vi "FindThetas.vi"(0 "strip":T3 {"a (cm)" format="%.2f"; "h (cm)" format="%.2f"; "radius (cm)" format="%.2f"}, 1 "r values (cm)":T5 {"r5" format="%.2f"; "r4" format="%.2f"; "r3" format="%.2f"; "r2" format="%.2f"; "r1" format="%.2f"; "r0" format="%.2f"}, 3 "Case Number":i32, 4 "Location Tests":T1, 5 "P constants":T4 {"Dtemp" format="%.2f"; "B" format="%.2f"; "A" format="%.2f"; "thetaw" format="%.2f"; "phih" format="%.2f"; "r (cm)" format="%.2f"}, 6 "Variables":T2={"sound spd (cm/s)"=150000, "time step (s)"=1e-09} {"time step (s)" format="%.2e"}, 7 "P (cm)":cluster{"x":dbl, "y":dbl, "z":dbl}={"x"=1.0, "y"=-5.0, "z"=2.0} {"x" format="%.2f"; "z" format="%.2f"; "y" format="%.2f"}) -> (8 "d":dbl[](array[numeric]) format="%.2f", 9 "min/max r":cluster{"max":dbl, "min":dbl} {"min" format="%.2f"; "max" format="%.2f"}, 10 "h(r,t) offset":dbl[](graph), 11 "cap to wedge offset":i32, 12 "h(r,t)":dbl[](graph), 13 "wedge delay pts":i32, 14 "beta(t)/2":dbl[](array[numeric]) format="%.2f", 15 "cap delay pts":i32, 17 "rmin out":dbl format="%.2f", 18 "sigma":dbl[](array[numeric]) format="%.2f", 19 "slice coords":dbl[][](array[numeric]) format="%.4f")   [LabVIEW 2022 SP3]
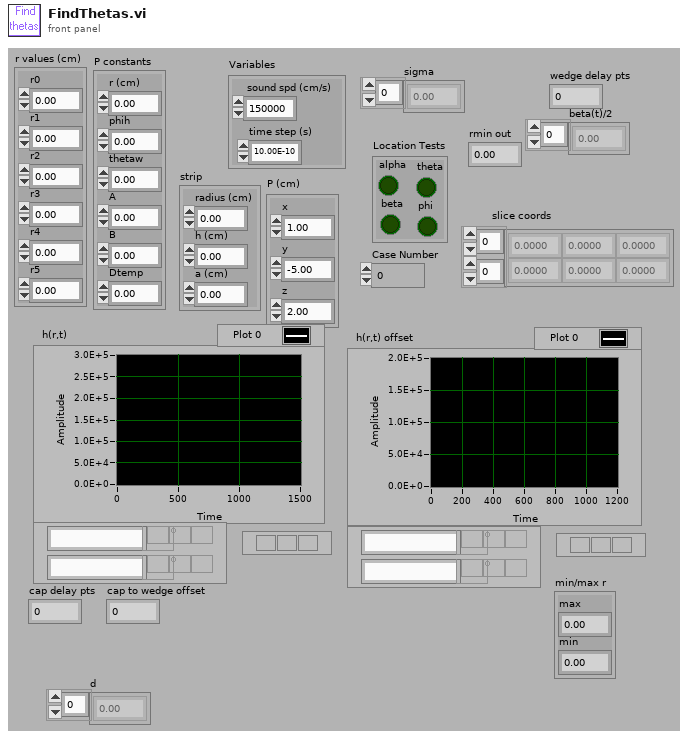
[diagram p1: front panel]
types:
  T1 = cluster{"alpha":bool, "beta":bool, "theta":bool, "phi":bool}
  T2 = cluster{"sound spd (cm/s)":i32, "time step (s)":sgl}
  T3 = cluster{"radius (cm)":dbl, "h (cm)":dbl, "a (cm)":dbl}
  T4 = cluster{"r (cm)":dbl, "phih":dbl, "thetaw":dbl, "A":dbl, "B":dbl, "Dtemp":dbl}
  T5 = cluster{"r0":dbl, "r1":dbl, "r2":dbl, "r3":dbl, "r4":dbl, "r5":dbl}
  T6 = cluster{"Number of rings":i32, "sound spd (cm/s)":i32, "z span (cm)":dbl, "z steps":i32, "y span (cm)":dbl, "y steps":i32, "time step (s)":sgl, "z":dbl, "y":dbl, "ref delay":dbl, "freq (MHz)":dbl, "cycles":i32}
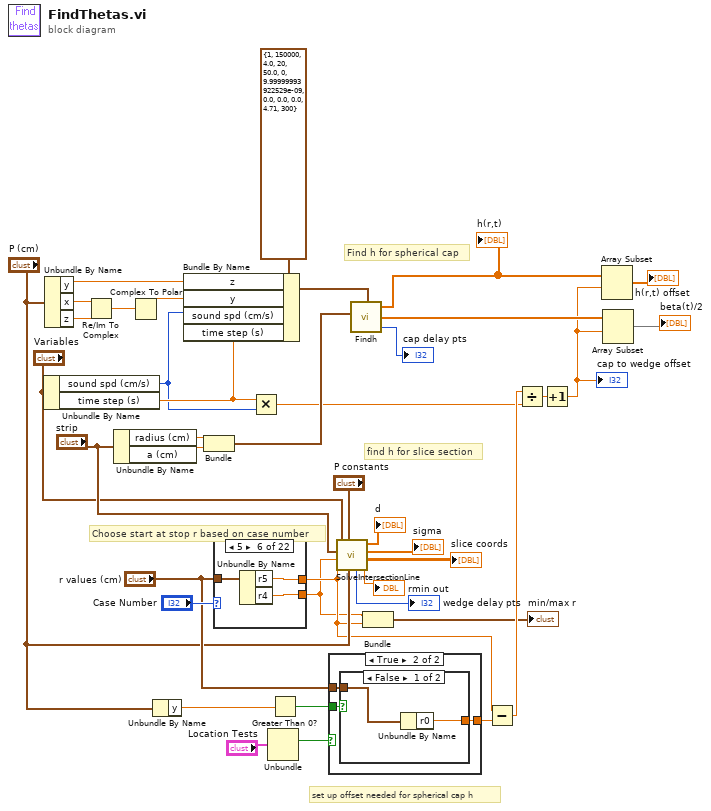
[diagram p0: block diagram]
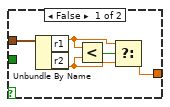
[diagram p2: hidden frame]
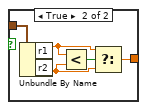
[diagram p3: hidden frame]
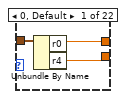
[diagram p4: hidden frame]
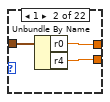
[diagram p5: hidden frame]
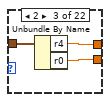
[diagram p6: hidden frame]
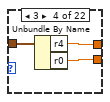
[diagram p7: hidden frame]
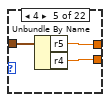
[diagram p8: hidden frame]
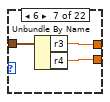
[diagram p9: hidden frame]
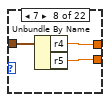
[diagram p10: hidden frame]
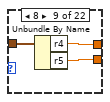
[diagram p11: hidden frame]
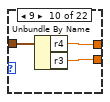
[diagram p12: hidden frame]
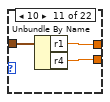
[diagram p13: hidden frame]
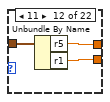
[diagram p14: hidden frame]
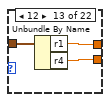
[diagram p15: hidden frame]
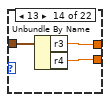
[diagram p16: hidden frame]
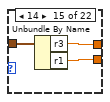
[diagram p17: hidden frame]
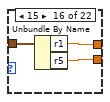
[diagram p18: hidden frame]
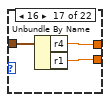
[diagram p19: hidden frame]
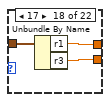
[diagram p20: hidden frame]
diagram:
  # "Find h for spherical cap"
  # "find h for slice section"
  # "set up offset needed for spherical cap h"
  # "Choose start at stop r based on case number"
  n1 = Unbundle By Name("Variables") -> ("sound spd (cm/s)"=w6:i32, "time step (s)"=w20:sgl)
  n2 = Unbundle By Name("P (cm)") -> ("y"=w17:dbl, "x"=w33:dbl, "z"=w32:dbl)
  n3 = Re/Im To Complex(1:w32, 2:w33) -> (0:w31:cdb)
  n4 = Unbundle By Name("strip") -> ("radius (cm)"=w36:dbl, "a (cm)"=w35:dbl)
  n5 = Complex To Polar(r * e^(i*theta)=w31) -> (r=w18:dbl)  [unwired: 1 out]
  n6 = Unbundle By Name("P (cm)") -> ("y"=w19:dbl)
  n7 = Bundle By Name(cluster=T6 {"Number of rings"=1, "sound spd (cm/s)"=150000, "z span (cm)"=4.0, "z steps"=20, "y span (cm)"=50.0, "y steps"=0, "time step (s)"=1e-08, "z"=0.0, "y"=0.0, "ref delay"=0.0, "freq (MHz)"=4.71, "cycles"=300} ("Variables in"), "z"=w17, "y"=w18, "sound spd (cm/s)"=w6, "time step (s)"=w20) -> (w38:T6)
  n8 = Bundle("radius (cm)"=w36, "a (cm)"=w35) -> (w34:cluster{"radius (cm)":dbl, "a (cm)":dbl})  [unwired: 1 out]
  n9 = case shown="5" "Case Number" {
    tunnel: "r values (cm)" -> [w41 w46 w49 w52 w55 w58 w61 w64 w67 w70 w73 w76 w79 w82 w85 w88 w91 w94 w97 w100 w103 w106]
    tunnel: [w43 w45 w48 w51 w54 w57 w60 w63 w66 w69 w72 w75 w78 w81 w84 w87 w90 w93 w96 w99 w102 w105] -> w4
    tunnel: [w42 w44 w47 w50 w53 w56 w59 w62 w65 w68 w71 w74 w77 w80 w83 w86 w89 w92 w95 w98 w101 w104] -> w3
    frame 0, Default {
      n10 = Unbundle By Name(w41) -> ("r0"=w43:dbl, "r4"=w42:dbl)
    }
    frame 1 {
      n11 = Unbundle By Name(w46) -> ("r0"=w45:dbl, "r4"=w44:dbl)
    }
    frame 2 {
      n12 = Unbundle By Name(w49) -> ("r4"=w48:dbl, "r0"=w47:dbl)
    }
    frame 3 {
      n13 = Unbundle By Name(w52) -> ("r4"=w51:dbl, "r0"=w50:dbl)
    }
    frame 4 {
      n14 = Unbundle By Name(w55) -> ("r5"=w54:dbl, "r4"=w53:dbl)
    }
    frame 5 {
      n15 = Unbundle By Name(w58) -> ("r5"=w57:dbl, "r4"=w56:dbl)
    }
    frame 6 {
      n16 = Unbundle By Name(w61) -> ("r3"=w60:dbl, "r4"=w59:dbl)
    }
    frame 7 {
      n17 = Unbundle By Name(w64) -> ("r4"=w63:dbl, "r5"=w62:dbl)
    }
    frame 8 {
      n18 = Unbundle By Name(w67) -> ("r4"=w66:dbl, "r5"=w65:dbl)
    }
    frame 9 {
      n19 = Unbundle By Name(w70) -> ("r4"=w69:dbl, "r3"=w68:dbl)
    }
    frame 10 {
      n20 = Unbundle By Name(w73) -> ("r1"=w72:dbl, "r4"=w71:dbl)
    }
    frame 11 {
      n21 = Unbundle By Name(w76) -> ("r5"=w75:dbl, "r1"=w74:dbl)
    }
    frame 12 {
      n22 = Unbundle By Name(w79) -> ("r1"=w78:dbl, "r4"=w77:dbl)
    }
    frame 13 {
      n23 = Unbundle By Name(w82) -> ("r3"=w81:dbl, "r4"=w80:dbl)
    }
    frame 14 {
      n24 = Unbundle By Name(w85) -> ("r3"=w84:dbl, "r1"=w83:dbl)
    }
    frame 15 {
      n25 = Unbundle By Name(w88) -> ("r1"=w87:dbl, "r5"=w86:dbl)
    }
    frame 16 {
      n26 = Unbundle By Name(w91) -> ("r4"=w90:dbl, "r1"=w89:dbl)
    }
    frame 17 {
      n27 = Unbundle By Name(w94) -> ("r1"=w93:dbl, "r3"=w92:dbl)
    }
    frame 18 {
      n28 = Unbundle By Name(w97) -> ("r4"=w96:dbl, "r3"=w95:dbl)
    }
    frame 19 {
      n29 = Unbundle By Name(w100) -> ("r4"=w99:dbl, "r1"=w98:dbl)
    }
    frame 20 {
      n30 = Unbundle By Name(w103) -> ("r5"=w102:dbl, "r1"=w101:dbl)
    }
    frame 21 {
      n31 = Unbundle By Name(w106) -> ("r1"=w105:dbl, "r5"=w104:dbl)
    }
  }
  n32 = Multiply(x=w20, y=w6) -> (x*y=w15:sgl)
  n33 = Unbundle("Location Tests") -> ("beta"=w24:bool)  [unwired: 3 out]
  n34 = Greater Than 0?(x=w19) -> (x > 0?=w22:bool)
  n35 = case shown="True" w24 {
    tunnel: "r values (cm)" -> [w110 w114]
    tunnel: [w111 w113] -> w21
    tunnel: w22 -> [_ w112]
    frame False {
      n36 = Unbundle By Name(w110) -> ("r1"=w109:dbl, "r2"=w108:dbl)
      n37 = Less?(x=w109, y=w108) -> (x < y?=w107:bool)
      n38 = Select(t=w109, s=w107, f=w108) -> (s? t:f=w111:dbl)
    }
    frame True {
      n39 = case shown="False" w112 {
        tunnel: w114 -> [w116 w118]
        tunnel: [w115 w117] -> w113
        frame False {
          n40 = Unbundle By Name(w116) -> ("r0"=w115:dbl)
        }
        frame True {
          n41 = Unbundle By Name(w118) -> ("r1"=w121:dbl, "r2"=w120:dbl)
          n42 = Less?(x=w121, y=w120) -> (x < y?=w119:bool)
          n43 = Select(t=w121, s=w119, f=w120) -> (s? t:f=w117:dbl)
        }
      }
    }
  }
  n44 = call "SolveIntersectionLine.vi"("P (cm)"="P (cm)", "P Variables"="P constants", "min"=w4, "max"=w3, "strip"="strip", "Variables"="Variables") -> ("rmin"=→"rmin out":dbl, "slice thetas"=→"slice coords":dbl[][], "sigma"=→"sigma":dbl[], "d"=→"d":dbl[], "wedge delay pts"=→"wedge delay pts":i32)  [unwired: 1 out]
  n45 = call "Findh.vi"("Trans Geometry"=w34, "Variables in"=w38) -> ("h(r,t)"=w5:dbl[], "beta(t)/2"=w25:dbl[], "delay pts"=→"cap delay pts":i32)  [unwired: 1 in, 2 out]
  "h(r,t)" <- w5
  n46 = Bundle("r5"=w3, "r1"=w4) -> (→"min/max r":cluster{"r5":dbl, "r1":dbl})  [unwired: 1 out]
  n47 = Subtract(x=w4, y=w21) -> (x-y=w16:dbl)
  n48 = Divide(x=w16, y=w15) -> (x/y=w11:dbl)
  n49 = Increment(x=w11) -> (x+1=w10:dbl)
  "cap to wedge offset" <- w10
  n50 = Array Subset(array=w5, index=w10) -> (→"h(r,t) offset":dbl[])  [unwired: 1 in]
  n51 = Array Subset(array=w25, index=w10) -> (→"beta(t)/2":dbl[])  [unwired: 1 in]
